vi "Handle Command.vi"(8 "error in (no error)":errorcluster, 9 "Value":bool, 11 "Valve in":refnum<class "BangBangControl.lvclass">) -> (0 "error out":errorcluster, 3 "Valve out":refnum<class "BangBangControl.lvclass">)   [LabVIEW 2020, in "VolatusControl.lvlib" / "BangBangControl.lvclass"]
uses:
  BangBangControl.lvclass
  State.ctl
  BangBangControl.lvclass/BangBangControl.ctl
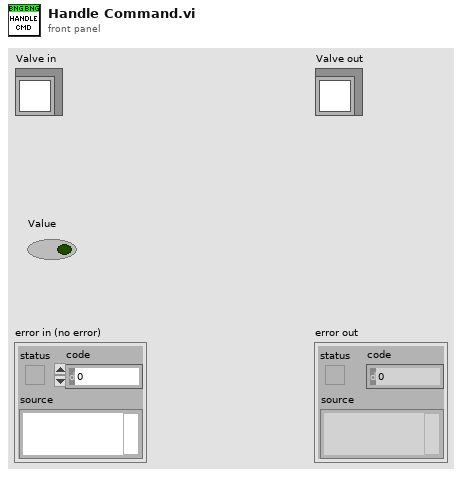
[diagram p1: front panel]
types:
  T1 = typedef "VolatusControl.lvlib/BangBangControl.lvclass/State.ctl" = enum16{"Idle", "RampUp", "RampDown", "Hold", "Disable", "Enable"}
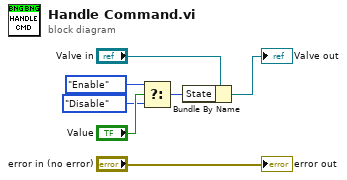
[diagram p0: block diagram]
diagram:
  n1 = Select(t=State."Enable" ("State"), s="Value", f=State."Disable" ("State")) -> (s? t:f=w1:T1)
  n2 = Bundle By Name(cluster="Valve in", "State"=w1) -> (→"Valve out":refnum<class "BangBangControl.lvclass">)
  "error out" <- "error in (no error)"
